vi "S4GUI_002.vi"(7 "Tab ObsEng":enum32{"Obs", "CCD modes", "Eng"}(tab)) -> ()   [LabVIEW 2018] (continued)
        n4615 = call "Write Instrument.lvclass.vi"("error in (no error)"=w11048, "Instrument.lvclass"=w11033, "S4ACS_GUI in"=w11035) -> ("error out"=w11029:errorcluster, "S4ACS_GUI out"=w11030:refnum<class "S4GUI.lvclass">)  [unwired: 7 in]
        n4616 = call "Read Instrument.lvclass.vi"("error in (no error)"=w11029, "S4ACS_GUI in"=w11030) -> ("error out"=w11098:errorcluster, "Instrument.lvclass"=w11099:refnum<class "Instrument.lvclass">, "S4ACS_GUI out"=w10945:refnum<class "S4GUI.lvclass">)  [unwired: 7 in]
        n4617 = call "Read WPSEL.vi"("error in (no error)"=w11098, "Instrument in"=w11099) -> ("error out"=w11095:errorcluster, "Opt_Selector.lvclass"=w11097:refnum<class "Opt_Selector.lvclass">, "Instrument out"=w11089:refnum<class "Instrument.lvclass">)  [unwired: 7 in]
        n4618 = call-dynamic "Read State Machine.vi"("error in (no error)"=w11095, "Device in"=w11097) -> ("error out"=w11094:errorcluster, "State Machine.lvclass"=w11087:refnum<class "State Machine.lvclass">, "Device out"=w11091:refnum<class "Opt_Selector.lvclass">)  [unwired: 7 in]
        n4619 = call "Next State.vi"("error in (no error)"=w11094, "New_State"=1, "State Machine in"=w11087) -> ("error out"=w11093:errorcluster, "State Machine out"=w11092:refnum<class "State Machine.lvclass">)  [unwired: 7 in]
        n4620 = call-dynamic "Write State Machine.vi"("error in (no error)"=w11093, "State Machine.lvclass"=w11092, "Device in"=w11091) -> ("error out"=w11088:errorcluster, "Device out"=w11090:refnum<class "Opt_Selector.lvclass">)  [unwired: 7 in]
        n4621 = call "Write WPSEL.vi"("error in (no error)"=w11088, "Opt_Selector.lvclass"=w11090, "Instrument in"=w11089) -> ("error out"=w11079:errorcluster, "Instrument out"=w11078:refnum<class "Instrument.lvclass">)  [unwired: 7 in]
        n4622 = call "Read ASEL.vi"("error in (no error)"=w11079, "Instrument in"=w11078) -> ("error out"=w11085:errorcluster, "Opt_Selector.lvclass"=w11076:refnum<class "Opt_Selector.lvclass">, "Instrument out"=w11077:refnum<class "Instrument.lvclass">)  [unwired: 7 in]
        n4623 = call-dynamic "Read State Machine.vi"("error in (no error)"=w11085, "Device in"=w11076) -> ("error out"=w11084:errorcluster, "State Machine.lvclass"=w11080:refnum<class "State Machine.lvclass">, "Device out"=w11075:refnum<class "Opt_Selector.lvclass">)  [unwired: 7 in]
        n4624 = call "Next State.vi"("error in (no error)"=w11084, "New_State"=1, "State Machine in"=w11080) -> ("error out"=w11083:errorcluster, "State Machine out"=w11082:refnum<class "State Machine.lvclass">)  [unwired: 7 in]
        n4625 = call-dynamic "Write State Machine.vi"("error in (no error)"=w11083, "State Machine.lvclass"=w11082, "Device in"=w11075) -> ("error out"=w11081:errorcluster, "Device out"=w11074:refnum<class "Opt_Selector.lvclass">)  [unwired: 7 in]
        n4626 = Concatenate Strings("SET WAVEPLATE:  WPSEL=" ("string"), w10924, " CALW=" ("string"), w10927) -> (w10937:string)
        n4627 = call "Write ASEL.vi"("error in (no error)"=w11081, "Opt_Selector.lvclass"=w11074, "Instrument in"=w11077) -> ("error out"=w11061:errorcluster, "Instrument out"=w11063:refnum<class "Instrument.lvclass">)  [unwired: 7 in]
        n4628 = call "Read CALW.vi"("error in (no error)"=w11061, "Instrument in"=w11063) -> ("error out"=w11071:errorcluster, "Opt_Selector.lvclass"=w11073:refnum<class "Opt_Selector.lvclass">, "Instrument out"=w11062:refnum<class "Instrument.lvclass">)  [unwired: 7 in]
        n4629 = call-dynamic "Read State Machine.vi"("error in (no error)"=w11071, "Device in"=w11073) -> ("error out"=w11070:errorcluster, "State Machine.lvclass"=w11064:refnum<class "State Machine.lvclass">, "Device out"=w11067:refnum<class "Opt_Selector.lvclass">)  [unwired: 7 in]
        n4630 = call "Next State.vi"("error in (no error)"=w11070, "New_State"=1, "State Machine in"=w11064) -> ("error out"=w11069:errorcluster, "State Machine out"=w11068:refnum<class "State Machine.lvclass">)  [unwired: 7 in]
        n4631 = call-dynamic "Write State Machine.vi"("error in (no error)"=w11069, "State Machine.lvclass"=w11068, "Device in"=w11067) -> ("error out"=w11065:errorcluster, "Device out"=w11066:refnum<class "Opt_Selector.lvclass">)  [unwired: 7 in]
        n4632 = property on="Lambda Selector" class="Ring (strict)"() -> ("RingText.Text"=w11060:string)  [unwired: 2 in, 2 out]
        n4633 = call "Write CALW.vi"("error in (no error)"=w11065, "Opt_Selector.lvclass"=w11066, "Instrument in"=w11062) -> ("error out"=w10944:errorcluster, "Instrument out"=w11059:refnum<class "Instrument.lvclass">)  [unwired: 7 in]
        n4634 = call-dynamic "Read mode EXPOSE.vi"("error in (no error)"=w10944, "S4GUI in"=w10945) -> ("error out"=w10943:errorcluster, "mode EXPOSE"=w10941:bool, "S4GUI out"=w10942:refnum<class "S4GUI.lvclass">)  [unwired: 7 in]
        n4635 = call-dynamic "Read sync.vi"("error in (no error)"=w10943, "S4ACS_GUI in"=w10942) -> ("error out"=w10961:errorcluster, "sync"=w10960:bool, "S4ACS_GUI out"=w10962:refnum<class "S4GUI.lvclass">)  [unwired: 7 in]
        n4636 = case shown="\"OFF\"" w11060 {
          selector: w11060 -> [w11307 _]
          tunnel: w11059 -> [w11311 w11329]
          tunnel: [w11310 w11329] -> w11058
          tunnel: [w11303 w11328] -> w10978
          tunnel: w10961 -> [w11309 w11328]
          tunnel: [w11300 w11324] -> w10973
          tunnel: w10960 -> [w11299 _]
          tunnel: w10941 -> [w11298 w11327]
          frame "OFF" {
            w11301 = u16 0 items=["OFF", "POLARIZER", "PINHOLE", "SHUTTER", "DEPOLARIZER"] ("Calibrator Selector 2")
            n4637 = call "Read CALW.vi"("error in (no error)"=w11309, "Instrument in"=w11311) -> ("error out"=w11314:errorcluster, "Opt_Selector.lvclass"=w11316:refnum<class "Opt_Selector.lvclass">, "Instrument out"=w11315:refnum<class "Instrument.lvclass">)  [unwired: 7 in]
            n4638 = call "Write target.vi"("error in (no error)"=w11314, "target"=0.0, "Optics in"=w11316) -> ("error out"=w11313:errorcluster, "Optics out"=w11317:refnum<class "Opt_Selector.lvclass">)  [unwired: 7 in]
            n4639 = call "Write target name.vi"("error in (no error)"=w11313, "target name"=w11307, "Optics in"=w11317) -> ("error out"=w11312:errorcluster, "Optics out"=w11318:refnum<class "Opt_Selector.lvclass">)  [unwired: 7 in]
            n4640 = call "Write CALW.vi"("error in (no error)"=w11312, "Opt_Selector.lvclass"=w11318, "Instrument in"=w11315) -> ("error out"=w11302:errorcluster, "Instrument out"=w11310:refnum<class "Instrument.lvclass">)  [unwired: 7 in]
            n4641 = property on="Calibrator Selector" class="Ring (strict)"(error in=w11302, "Value"=w11301, "DisabledEnum"=T12."Disabled and Grayed Out" ("Disabled")) -> (error out=w11304:errorcluster)  [unwired: 1 in, 1 out]
            n4642 = property on="Calibrator Selector" class="Ring (strict)"(error in=w11304, "RingText.Text"="OFF" ("Ring Text.Text")) -> (error out=w11303:errorcluster)  [unwired: 1 in, 1 out]
            n4643 = case shown="True" w11299 {
              tunnel: [u8 0 ("SHUTTER_MODE") w11321] -> w11300
              tunnel: w11298 -> [_ w11320]
              frame False {
                # "Fotom. & Async"
                # "Internal"
              }
              frame True {
                # "Ext. Start"
                # "Internal"
                # "Fotom. Sync. SEM exp mode"
                # "Fotom. Sync. COM exp mode"
                n4644 = Select(t=u8 0, s=w11320, f=u8 6 ("SHUTTER_MODE")) -> (s? t:f=w11321:u8)
              }
            }
          }
          frame Default {
            # "Polar. COM exp mode"
            # "Internal"
            # "Polar. SEM exp mode"
            # "Ext. Start"
            n4645 = Select(t=u8 0, s=w11327, f=u8 6 ("SHUTTER_MODE")) -> (s? t:f=w11324:u8)
          }
        }
        n4646 = call "Write Instrument.lvclass.vi"("error in (no error)"=w10978, "Instrument.lvclass"=w11058, "S4ACS_GUI in"=w10962) -> ("error out"=w10977:errorcluster, "S4ACS_GUI out"=w10966:refnum<class "S4GUI.lvclass">)  [unwired: 7 in]
        n4647 = call-dynamic "Read AcquisitionC.vi"("error in (no error)"=w10977, "S4ACS_GUI in"=w10966) -> ("error out"=w10988:errorcluster, "Acquisition.lvclass"=w10987:refnum<class "Acquisition.lvclass">)  [unwired: 7 in, 1 out]
        n4648 = call-dynamic "Read AcquisitionA.vi"("error in (no error)"=w10977, "S4ACS_GUI in"=w10966) -> ("error out"=w10991:errorcluster, "Acquisition.lvclass"=w10992:refnum<class "Acquisition.lvclass">)  [unwired: 7 in, 1 out]
        n4649 = call "Read AcquisitionB.vi"("error in (no error)"=w10977, "S4ACS_GUI in"=w10966) -> ("error out"=w10989:errorcluster, "Acquisition.lvclass"=w10990:refnum<class "Acquisition.lvclass">)  [unwired: 7 in, 1 out]
        n4650 = call-dynamic "Read AcquisitionD.vi"("error in (no error)"=w10977, "S4ACS_GUI in"=w10966) -> ("error out"=w10985:errorcluster, "Acquisition.lvclass"=w10986:refnum<class "Acquisition.lvclass">)  [unwired: 7 in, 1 out]
        n4651 = call "Read connection.vi"("error in (no error)"=w10988, "Server in"=w10987) -> ("error out"=w10994:errorcluster, "connection"=w10993:bool, "Server out"=w10995:refnum<class "Acquisition.lvclass">)  [unwired: 7 in]
        n4652 = call "Read connection.vi"("error in (no error)"=w10989, "Server in"=w10990) -> ("error out"=w10997:errorcluster, "connection"=w10996:bool, "Server out"=w10998:refnum<class "Acquisition.lvclass">)  [unwired: 7 in]
        n4653 = call "Read connection.vi"("error in (no error)"=w10985, "Server in"=w10986) -> ("error out"=w10974:errorcluster, "connection"=w10975:bool, "Server out"=w10976:refnum<class "Acquisition.lvclass">)  [unwired: 7 in]
        n4654 = call "Read connection.vi"("error in (no error)"=w10991, "Server in"=w10992) -> ("error out"=w11000:errorcluster, "connection"=w10999:bool, "Server out"=w11001:refnum<class "Acquisition.lvclass">)  [unwired: 7 in]
        n4655 = case shown="True" w10993 {
          tunnel: w10995 -> [w11165 w11170]
          tunnel: w10994 -> [w11164 w11169]
          tunnel: [w11165 w11168] -> w10980
          tunnel: [w11164 w11167] -> w10979
          tunnel: w10973 -> [_ w11166]
          frame False {
          }
          frame True {
            # "nome do arquivo .cfg"
            # "seção no arquivo .cfg"
            n4656 = call-dynamic "Read Channel.vi"("error in (no error)"=w11169, "Acquisition in"=w11170) -> ("error out"=w11174:errorcluster, "Channel.lvclass"=w11173:refnum<class "Channel.lvclass">, "Acquisition out"=w11172:refnum<class "Acquisition.lvclass">)  [unwired: 7 in]
            n4657 = call-dynamic "Read Interface.vi"("error in (no error)"=w11174, "Channel in"=w11173) -> ("error out"=w11181:errorcluster, "Interface.lvclass"=w11182:refnum<class "Interface.lvclass">, "Channel out"=w11171:refnum<class "Channel.lvclass">)  [unwired: 7 in]
            n4658 = call-dynamic "Get CCD_Config.vi"("error in (no error)"=w11181, "Interface in"=w11182) -> ("error out"=w11179:errorcluster, "output cluster"=w11178:T31, "Interface out"=w11183:refnum<class "Interface.lvclass">)  [unwired: 7 in]
            n4659 = Bundle By Name(cluster=w11178, "TRIGGER_MODE"=w11166) -> (w11180:T31)
            n4660 = call-dynamic "Set CCD_Config.vi"("error in (no error)"=w11179, "input cluster"=w11180, "Interface in"=w11183) -> ("error out"=w11177:errorcluster, "Interface out"=w11184:refnum<class "Interface.lvclass">)  [unwired: 7 in]
            n4661 = Flatten To String(anything=w11180, error in (no error)=w11177) -> (data string=w11175:string, error out=w11176:errorcluster)  [unwired: 2 in, 1 out]
            n4662 = call "Write flatted cluster.vi"("error in (no error)"=w11176, "flatted cluster"=w11175, "Interface in"=w11184) -> ("error out"=w11186:errorcluster, "Interface out"=w11185:refnum<class "Interface.lvclass">)  [unwired: 7 in]
            n4663 = call-dynamic "Write Interface.vi"("error in (no error)"=w11186, "Interface.lvclass"=w11185, "Channel in"=w11171) -> ("error out"=w11192:errorcluster, "Channel out"=w11193:refnum<class "Channel.lvclass">)  [unwired: 7 in]
            n4664 = call "Write section_name.vi"("error in (no error)"=w11192, "section_name"="CCD_ACS3", "Channel in"=w11193) -> ("error out"=w11190:errorcluster, "Channel out"=w11196:refnum<class "Channel.lvclass">)  [unwired: 7 in]
            n4665 = call-dynamic "save config.vi"("error in (no error)"=w11190, "file config"="lastsaved.cfg", "Channel in"=w11196) -> ("error out"=w11191:errorcluster, "Channel out"=w11197:refnum<class "Channel.lvclass">)  [unwired: 7 in]
            n4666 = call-dynamic "Read State Machine.vi"("error in (no error)"=w11191, "Device in"=w11197) -> ("error out"=w11187:errorcluster, "State Machine.lvclass"=w11199:refnum<class "State Machine.lvclass">, "Device out"=w11198:refnum<class "Channel.lvclass">)  [unwired: 7 in]
            n4667 = call-dynamic "Write State.vi"("error in (no error)"=w11187, "State"=60, "State Machine in"=w11199) -> ("error out"=w11188:errorcluster, "State Machine out"=w11200:refnum<class "State Machine.lvclass">)  [unwired: 7 in]
            n4668 = call-dynamic "Write State Machine.vi"("error in (no error)"=w11188, "State Machine.lvclass"=w11200, "Device in"=w11198) -> ("error out"=w11202:errorcluster, "Device out"=w11201:refnum<class "Channel.lvclass">)  [unwired: 7 in]
            n4669 = call-dynamic "Write Channel.vi"("error in (no error)"=w11202, "Channel.lvclass"=w11201, "Acquisition in"=w11172) -> ("error out"=w11167:errorcluster, "Acquisition out"=w11168:refnum<class "Acquisition.lvclass">)  [unwired: 7 in]
          }
        }
        n4670 = case shown="True" w10975 {
          tunnel: w10976 -> [w11126 w11131]
          tunnel: w10974 -> [w11125 w11130]
          tunnel: w10973 -> [_ w11129]
          tunnel: [w11126 w11128] -> w10972
          tunnel: [w11125 w11127] -> w10971
          frame False {
          }
          frame True {
            # "nome do arquivo .cfg"
            # "seção no arquivo .cfg"
            n4671 = call-dynamic "Read Channel.vi"("error in (no error)"=w11130, "Acquisition in"=w11131) -> ("error out"=w11160:errorcluster, "Channel.lvclass"=w11161:refnum<class "Channel.lvclass">, "Acquisition out"=w11162:refnum<class "Acquisition.lvclass">)  [unwired: 7 in]
            n4672 = call-dynamic "Read Interface.vi"("error in (no error)"=w11160, "Channel in"=w11161) -> ("error out"=w11153:errorcluster, "Interface.lvclass"=w11152:refnum<class "Interface.lvclass">, "Channel out"=w11163:refnum<class "Channel.lvclass">)  [unwired: 7 in]
            n4673 = call-dynamic "Get CCD_Config.vi"("error in (no error)"=w11153, "Interface in"=w11152) -> ("error out"=w11155:errorcluster, "output cluster"=w11156:T31, "Interface out"=w11151:refnum<class "Interface.lvclass">)  [unwired: 7 in]
            n4674 = Bundle By Name(cluster=w11156, "TRIGGER_MODE"=w11129) -> (w11154:T31)
            n4675 = call-dynamic "Set CCD_Config.vi"("error in (no error)"=w11155, "input cluster"=w11154, "Interface in"=w11151) -> ("error out"=w11157:errorcluster, "Interface out"=w11150:refnum<class "Interface.lvclass">)  [unwired: 7 in]
            n4676 = Flatten To String(anything=w11154, error in (no error)=w11157) -> (data string=w11159:string, error out=w11158:errorcluster)  [unwired: 2 in, 1 out]
            n4677 = call "Write flatted cluster.vi"("error in (no error)"=w11158, "flatted cluster"=w11159, "Interface in"=w11150) -> ("error out"=w11148:errorcluster, "Interface out"=w11149:refnum<class "Interface.lvclass">)  [unwired: 7 in]
            n4678 = call-dynamic "Write Interface.vi"("error in (no error)"=w11148, "Interface.lvclass"=w11149, "Channel in"=w11163) -> ("error out"=w11142:errorcluster, "Channel out"=w11141:refnum<class "Channel.lvclass">)  [unwired: 7 in]
            n4679 = call "Write section_name.vi"("error in (no error)"=w11142, "section_name"="CCD_ACS4", "Channel in"=w11141) -> ("error out"=w11144:errorcluster, "Channel out"=w11138:refnum<class "Channel.lvclass">)  [unwired: 7 in]
            n4680 = call-dynamic "save config.vi"("error in (no error)"=w11144, "file config"="lastsaved.cfg", "Channel in"=w11138) -> ("error out"=w11143:errorcluster, "Channel out"=w11137:refnum<class "Channel.lvclass">)  [unwired: 7 in]
            n4681 = call-dynamic "Read State Machine.vi"("error in (no error)"=w11143, "Device in"=w11137) -> ("error out"=w11147:errorcluster, "State Machine.lvclass"=w11135:refnum<class "State Machine.lvclass">, "Device out"=w11136:refnum<class "Channel.lvclass">)  [unwired: 7 in]
            n4682 = call-dynamic "Write State.vi"("error in (no error)"=w11147, "State"=60, "State Machine in"=w11135) -> ("error out"=w11146:errorcluster, "State Machine out"=w11134:refnum<class "State Machine.lvclass">)  [unwired: 7 in]
            n4683 = call-dynamic "Write State Machine.vi"("error in (no error)"=w11146, "State Machine.lvclass"=w11134, "Device in"=w11136) -> ("error out"=w11132:errorcluster, "Device out"=w11133:refnum<class "Channel.lvclass">)  [unwired: 7 in]
            n4684 = call-dynamic "Write Channel.vi"("error in (no error)"=w11132, "Channel.lvclass"=w11133, "Acquisition in"=w11162) -> ("error out"=w11127:errorcluster, "Acquisition out"=w11128:refnum<class "Acquisition.lvclass">)  [unwired: 7 in]
          }
        }
        n4685 = case shown="True" w10996 {
          tunnel: w10998 -> [w11204 w11209]
          tunnel: w10997 -> [w11203 w11208]
          tunnel: [w11204 w11207] -> w10982
          tunnel: [w11203 w11206] -> w10981
          tunnel: w10973 -> [_ w11205]
          frame False {
          }
          frame True {
            # "nome do arquivo .cfg"
            # "seção no arquivo .cfg"
            n4686 = call-dynamic "Read Channel.vi"("error in (no error)"=w11208, "Acquisition in"=w11209) -> ("error out"=w11213:errorcluster, "Channel.lvclass"=w11212:refnum<class "Channel.lvclass">, "Acquisition out"=w11211:refnum<class "Acquisition.lvclass">)  [unwired: 7 in]
            n4687 = call-dynamic "Read Interface.vi"("error in (no error)"=w11213, "Channel in"=w11212) -> ("error out"=w11220:errorcluster, "Interface.lvclass"=w11221:refnum<class "Interface.lvclass">, "Channel out"=w11210:refnum<class "Channel.lvclass">)  [unwired: 7 in]
            n4688 = call-dynamic "Get CCD_Config.vi"("error in (no error)"=w11220, "Interface in"=w11221) -> ("error out"=w11218:errorcluster, "output cluster"=w11217:T31, "Interface out"=w11222:refnum<class "Interface.lvclass">)  [unwired: 7 in]
            n4689 = Bundle By Name(cluster=w11217, "TRIGGER_MODE"=w11205) -> (w11219:T31)
            n4690 = call-dynamic "Set CCD_Config.vi"("error in (no error)"=w11218, "input cluster"=w11219, "Interface in"=w11222) -> ("error out"=w11216:errorcluster, "Interface out"=w11223:refnum<class "Interface.lvclass">)  [unwired: 7 in]
            n4691 = Flatten To String(anything=w11219, error in (no error)=w11216) -> (data string=w11214:string, error out=w11215:errorcluster)  [unwired: 2 in, 1 out]
            n4692 = call "Write flatted cluster.vi"("error in (no error)"=w11215, "flatted cluster"=w11214, "Interface in"=w11223) -> ("error out"=w11225:errorcluster, "Interface out"=w11224:refnum<class "Interface.lvclass">)  [unwired: 7 in]
            n4693 = call-dynamic "Write Interface.vi"("error in (no error)"=w11225, "Interface.lvclass"=w11224, "Channel in"=w11210) -> ("error out"=w11231:errorcluster, "Channel out"=w11232:refnum<class "Channel.lvclass">)  [unwired: 7 in]
            n4694 = call "Write section_name.vi"("error in (no error)"=w11231, "section_name"="CCD_ACS2", "Channel in"=w11232) -> ("error out"=w11229:errorcluster, "Channel out"=w11235:refnum<class "Channel.lvclass">)  [unwired: 7 in]
            n4695 = call-dynamic "save config.vi"("error in (no error)"=w11229, "file config"="lastsaved.cfg", "Channel in"=w11235) -> ("error out"=w11230:errorcluster, "Channel out"=w11236:refnum<class "Channel.lvclass">)  [unwired: 7 in]
            n4696 = call-dynamic "Read State Machine.vi"("error in (no error)"=w11230, "Device in"=w11236) -> ("error out"=w11226:errorcluster, "State Machine.lvclass"=w11238:refnum<class "State Machine.lvclass">, "Device out"=w11237:refnum<class "Channel.lvclass">)  [unwired: 7 in]
            n4697 = call-dynamic "Write State.vi"("error in (no error)"=w11226, "State"=60, "State Machine in"=w11238) -> ("error out"=w11227:errorcluster, "State Machine out"=w11239:refnum<class "State Machine.lvclass">)  [unwired: 7 in]
            n4698 = call-dynamic "Write State Machine.vi"("error in (no error)"=w11227, "State Machine.lvclass"=w11239, "Device in"=w11237) -> ("error out"=w11241:errorcluster, "Device out"=w11240:refnum<class "Channel.lvclass">)  [unwired: 7 in]
            n4699 = call-dynamic "Write Channel.vi"("error in (no error)"=w11241, "Channel.lvclass"=w11240, "Acquisition in"=w11211) -> ("error out"=w11206:errorcluster, "Acquisition out"=w11207:refnum<class "Acquisition.lvclass">)  [unwired: 7 in]
          }
        }
        n4700 = case shown="True" w10999 {
          tunnel: [w11242 w11276] -> w10983
          tunnel: [w11243 w11275] -> w10984
          tunnel: w11001 -> [w11243 w11246]
          tunnel: w11000 -> [w11242 w11245]
          tunnel: w10973 -> [_ w11244]
          frame False {
          }
          frame True {
            # "nome do arquivo .cfg"
            # "seção no arquivo .cfg"
            n4701 = call-dynamic "Read Channel.vi"("error in (no error)"=w11245, "Acquisition in"=w11246) -> ("error out"=w11277:errorcluster, "Channel.lvclass"=w11278:refnum<class "Channel.lvclass">, "Acquisition out"=w11279:refnum<class "Acquisition.lvclass">)  [unwired: 7 in]
            n4702 = call-dynamic "Read Interface.vi"("error in (no error)"=w11277, "Channel in"=w11278) -> ("error out"=w11268:errorcluster, "Interface.lvclass"=w11267:refnum<class "Interface.lvclass">, "Channel out"=w11280:refnum<class "Channel.lvclass">)  [unwired: 7 in]
            n4703 = call-dynamic "Get CCD_Config.vi"("error in (no error)"=w11268, "Interface in"=w11267) -> ("error out"=w11270:errorcluster, "output cluster"=w11271:T31, "Interface out"=w11266:refnum<class "Interface.lvclass">)  [unwired: 7 in]
            n4704 = Bundle By Name(cluster=w11271, "TRIGGER_MODE"=w11244) -> (w11269:T31)
            n4705 = call-dynamic "Set CCD_Config.vi"("error in (no error)"=w11270, "input cluster"=w11269, "Interface in"=w11266) -> ("error out"=w11272:errorcluster, "Interface out"=w11265:refnum<class "Interface.lvclass">)  [unwired: 7 in]
            n4706 = Flatten To String(anything=w11269, error in (no error)=w11272) -> (data string=w11274:string, error out=w11273:errorcluster)  [unwired: 2 in, 1 out]
            n4707 = call "Write flatted cluster.vi"("error in (no error)"=w11273, "flatted cluster"=w11274, "Interface in"=w11265) -> ("error out"=w11263:errorcluster, "Interface out"=w11264:refnum<class "Interface.lvclass">)  [unwired: 7 in]
            n4708 = call-dynamic "Write Interface.vi"("error in (no error)"=w11263, "Interface.lvclass"=w11264, "Channel in"=w11280) -> ("error out"=w11258:errorcluster, "Channel out"=w11257:refnum<class "Channel.lvclass">)  [unwired: 7 in]
            n4709 = call "Write section_name.vi"("error in (no error)"=w11258, "section_name"="CCD_ACS1", "Channel in"=w11257) -> ("error out"=w11259:errorcluster, "Channel out"=w11254:refnum<class "Channel.lvclass">)  [unwired: 7 in]
            n4710 = call-dynamic "save config.vi"("error in (no error)"=w11259, "file config"="lastsaved.cfg", "Channel in"=w11254) -> ("error out"=w11247:errorcluster, "Channel out"=w11248:refnum<class "Channel.lvclass">)  [unwired: 7 in]
            n4711 = call-dynamic "Read State Machine.vi"("error in (no error)"=w11247, "Device in"=w11248) -> ("error out"=w11262:errorcluster, "State Machine.lvclass"=w11252:refnum<class "State Machine.lvclass">, "Device out"=w11253:refnum<class "Channel.lvclass">)  [unwired: 7 in]
            n4712 = call-dynamic "Write State.vi"("error in (no error)"=w11262, "State"=60, "State Machine in"=w11252) -> ("error out"=w11261:errorcluster, "State Machine out"=w11251:refnum<class "State Machine.lvclass">)  [unwired: 7 in]
            n4713 = call-dynamic "Write State Machine.vi"("error in (no error)"=w11261, "State Machine.lvclass"=w11251, "Device in"=w11253) -> ("error out"=w11249:errorcluster, "Device out"=w11250:refnum<class "Channel.lvclass">)  [unwired: 7 in]
            n4714 = call-dynamic "Write Channel.vi"("error in (no error)"=w11249, "Channel.lvclass"=w11250, "Acquisition in"=w11279) -> ("error out"=w11276:errorcluster, "Acquisition out"=w11275:refnum<class "Acquisition.lvclass">)  [unwired: 7 in]
          }
        }
        n4715 = call-dynamic "Write AcquisitionA.vi"("error in (no error)"=w10983, "Acquisition.lvclass"=w10984, "S4ACS_GUI in"=w10966) -> ("error out"=w10970:errorcluster, "S4ACS_GUI out"=w10965:refnum<class "S4GUI.lvclass">)  [unwired: 7 in]
        n4716 = call "Write AcquisitionB.vi"("error in (no error)"=w10981, "Acquisition.lvclass"=w10982, "S4ACS_GUI in"=w10965) -> ("error out"=w10969:errorcluster, "S4ACS_GUI out"=w10964:refnum<class "S4GUI.lvclass">)  [unwired: 7 in]
        n4717 = call-dynamic "Write AcquisitionC.vi"("error in (no error)"=w10979, "Acquisition.lvclass"=w10980, "S4ACS_GUI in"=w10964) -> ("error out"=w10968:errorcluster, "S4ACS_GUI out"=w10963:refnum<class "S4GUI.lvclass">)  [unwired: 7 in]
        n4718 = call-dynamic "Write AcquisitionD.vi"("error in (no error)"=w10971, "Acquisition.lvclass"=w10972, "S4ACS_GUI in"=w10963) -> ("error out"=w10967:errorcluster, "S4ACS_GUI out"=w10947:refnum<class "S4GUI.lvclass">)  [unwired: 7 in]
        n4719 = Merge Errors(w10970, w10969, w10968, w10967) -> (w10946:errorcluster)
        n4720 = call "Read Instrument.lvclass.vi"("error in (no error)"=w10946, "S4ACS_GUI in"=w10947) -> ("error out"=w10952:errorcluster, "Instrument.lvclass"=w10951:refnum<class "Instrument.lvclass">, "S4ACS_GUI out"=w10948:refnum<class "S4GUI.lvclass">)  [unwired: 7 in]
        n4721 = call "Read ASEL.vi"("error in (no error)"=w10952, "Instrument in"=w10951) -> ("error out"=w10959:errorcluster, "Opt_Selector.lvclass"=w10958:refnum<class "Opt_Selector.lvclass">, "Instrument out"=w10957:refnum<class "Instrument.lvclass">)  [unwired: 7 in]
        n4722 = call "Read target name.vi"("error in (no error)"=w10959, "Optics in"=w10958) -> ("error out"=w10955:errorcluster, "target name"=w10935:string, "Optics out"=w10956:refnum<class "Opt_Selector.lvclass">)  [unwired: 7 in]
        n4723 = call "Write ASEL.vi"("error in (no error)"=w10955, "Opt_Selector.lvclass"=w10956, "Instrument in"=w10957) -> ("error out"=w10954:errorcluster, "Instrument out"=w10950:refnum<class "Instrument.lvclass">)  [unwired: 7 in]
        n4724 = Concatenate Strings(w10937, " ASEL=" ("string"), w10935) -> (w10932:string)
        n4725 = case shown="\"ON\"" w10935 {
          tunnel: w10954 -> [w11101 w11112]
          tunnel: [w11101 w11108] -> w10953
          tunnel: w10950 -> [w11100 w11113]
          tunnel: [w11100 w11109] -> w10949
          frame Default {
          }
          frame "ON" {
            n4726 = call "Read WPROT.vi"("error in (no error)"=w11112, "Instrument in"=w11113) -> ("error out"=w11104:errorcluster, "Opt_Selector.lvclass"=w11111:refnum<class "Opt_Selector.lvclass">, "Instrument out"=w11110:refnum<class "Instrument.lvclass">)  [unwired: 7 in]
            n4727 = call-dynamic "Read sequencia.vi"("error in (no error)"=w11104, "Opt_Selector in"=w11111) -> ("error out"=w11103:errorcluster, "sequencia"=w11107:u16, "Opt_Selector out"=w11106:refnum<class "Opt_Selector.lvclass">)  [unwired: 7 in]
            n4728 = case shown="0" w11107 {
              tunnel: w11106 -> [w11115 w11124]
              tunnel: [w11115 w11120] -> w11105
              tunnel: w11103 -> [w11114 w11123]
              tunnel: [w11114 w11118] -> w11102
              frame Default {
              }
              frame 0 {
                n4729 = call-dynamic "Write sequencia.vi"("error in (no error)"=w11123, "sequencia"=u16 1, "Opt_Selector in"=w11124) -> ("error out"=w11119:errorcluster, "Opt_Selector out"=w11121:refnum<class "Opt_Selector.lvclass">)  [unwired: 7 in]
                n4730 = local write "P0"(TRUE ("P0")) -> ()
                n4731 = call-dynamic "Write sequencia_ant.vi"("error in (no error)"=w11119, "sequencia_ant"=u16 1, "Opt_Selector in"=w11121) -> ("error out"=w11118:errorcluster, "Opt_Selector out"=w11120:refnum<class "Opt_Selector.lvclass">)  [unwired: 7 in]
              }
            }
            n4732 = call "Write WPROT.vi"("error in (no error)"=w11102, "Opt_Selector.lvclass"=w11105, "Instrument in"=w11110) -> ("error out"=w11108:errorcluster, "Instrument out"=w11109:refnum<class "Instrument.lvclass">)  [unwired: 7 in]
          }
        }
        n4733 = call "Write Instrument.lvclass.vi"("error in (no error)"=w10953, "Instrument.lvclass"=w10949, "S4ACS_GUI in"=w10948) -> ("error out"=w10933:errorcluster, "S4ACS_GUI out"=w10934:refnum<class "S4GUI.lvclass">)  [unwired: 7 in]
        n4734 = call-dynamic "Write User Event.vi"("error in (no error)"=w10933, "User Event"=w10932, "S4GUI in"=w10934) -> ("error out"=w10930:errorcluster, "S4GUI out"=w10931:refnum<class "S4GUI.lvclass">)  [unwired: 7 in]
      }
      event "Init mode": Value Change {
        n4735 = event-data() -> ()  [unwired: 1 in, 4 out]
        n4736 = call-dynamic "Write User Event.vi"("error in (no error)"=w11333, "User Event"="INIT INSTRUMENT CLICKED", "S4GUI in"=w11334) -> ("error out"=w11331:errorcluster, "S4GUI out"=w11332:refnum<class "S4GUI.lvclass">)  [unwired: 7 in]
        n4737 = call-dynamic "Read Obs_state.vi"("error in (no error)"=w11331, "S4ACS_GUI in"=w11332) -> ("error out"=w11335:errorcluster, "Obs_state"=w11337:u32, "S4ACS_GUI out"=w11338:refnum<class "S4GUI.lvclass">)  [unwired: 7 in]
        n4738 = In Range and Coerce(upper limit=u32 226, x=w11337, lower limit=u32 220 ("upper limit")) -> (In Range?=w11336:bool)  [unwired: 1 out]
        n4739 = case shown="True" w11336 {
          tunnel: [w11346 w11354] -> w11342
          tunnel: [w11345 w11352] -> w11341
          tunnel: w11335 -> [w11344 w11353]
          tunnel: w11338 -> [w11343 w11355]
          frame False {
            n4740 = call-dynamic "Write sync.vi"("error in (no error)"=w11344, "sync"=TRUE, "S4ACS_GUI in"=w11343) -> ("error out"=w11348:errorcluster, "S4ACS_GUI out"=w11347:refnum<class "S4GUI.lvclass">)  [unwired: 7 in]
            n4741 = call-dynamic "Write Obs_state.vi"("error in (no error)"=w11348, "Obs_state"=u32 220, "S4ACS_GUI in"=w11347) -> ("error out"=w11345:errorcluster, "S4ACS_GUI out"=w11346:refnum<class "S4GUI.lvclass">)  [unwired: 7 in]
          }
          frame True {
            n4742 = call-dynamic "Write Obs_state.vi"("error in (no error)"=w11353, "Obs_state"=u32 0, "S4ACS_GUI in"=w11355) -> ("error out"=w11352:errorcluster, "S4ACS_GUI out"=w11354:refnum<class "S4GUI.lvclass">)  [unwired: 7 in]
          }
        }
      }
      event "exit": Value Change {
        n4743 = event-data() -> ()  [unwired: 1 in, 4 out]
        n4744 = call-dynamic "Read Obs_state.vi"("error in (no error)"=w11359, "S4ACS_GUI in"=w11360) -> ("error out"=w11357:errorcluster, "Obs_state"=w11361:u32, "S4ACS_GUI out"=w11358:refnum<class "S4GUI.lvclass">)  [unwired: 7 in]
        n4745 = In Range and Coerce(upper limit=u32 239, x=w11361, lower limit=u32 230 ("upper limit")) -> (In Range?=w11356:bool)  [unwired: 1 out]
        n4746 = case shown="False" w11356 {
          tunnel: [w11374 w11494] -> w11365
          tunnel: [w11373 w11493] -> w11364
          tunnel: w11358 -> [w11367 w11494]
          tunnel: w11357 -> [w11366 w11493]
          frame False {
            n4747 = call "Read Instrument.lvclass.vi"("error in (no error)"=w11366, "S4ACS_GUI in"=w11367) -> ("error out"=w11368:errorcluster, "Instrument.lvclass"=w11370:refnum<class "Instrument.lvclass">, "S4ACS_GUI out"=w11372:refnum<class "S4GUI.lvclass">)  [unwired: 7 in]
            n4748 = call-dynamic "Read operational.vi"("error in (no error)"=w11368, "Server in"=w11370) -> ("error out"=w11371:errorcluster, "operational"=w11369:bool)  [unwired: 7 in, 1 out]
            n4749 = case shown="False" w11369 {
              tunnel: [w11381 w11438] -> w11374
              tunnel: [w11380 w11437] -> w11373
              tunnel: w11372 -> [w11376 w11440]
              tunnel: w11371 -> [w11375 w11439]
              frame False {
                # "S4ICS not operational: only ACS parking can \nbe allowed, depending on its status..."
                n4750 = call-dynamic "VerifyAcqStatus.vi"("error in (no error)"=w11375, "S4GUI in"=w11376) -> ("error out"=w11377:errorcluster, "idle"=w11379:bool, "S4GUI out"=w11378:refnum<class "S4GUI.lvclass">)  [unwired: 6 in, 1 out]
                n4751 = case shown="True" w11379 {
                  tunnel: w11377 -> [w11390 w11409]
                  tunnel: w11378 -> [w11391 w11408]
                  tunnel: [w11384 w11407] -> w11381
                  tunnel: [w11383 w11406] -> w11380
                  frame False {
                    # "Acquisition in progress..."
                    n4752 = Two Button Dialog(message="Parking not possible.\nAre you sure to quit?", 2:"Yes" ("T button name (\"OK\")")) -> (T button?=w11387:bool)  [unwired: 1 in]
                    n4753 = case shown="False" w11387 {
                      tunnel: [w11394 w11398] -> w11386
                      tunnel: w11391 -> [w11394 w11399]
                      tunnel: w11390 -> [w11393 w11397]
                      tunnel: [w11393 w11396] -> w11385
                      tunnel: ["EXIT CLICKED \nWITH NO PARKING \nPOSSIBLE. EXIT\nCANCELLED. " ("T button name (\"OK\")") "EXIT CLICKED WITH\nNO PARKING POSSIBLE. EXIT" ("T button name (\"OK\")")] -> w11382
                      frame False {
                        # "NO (cancel)"
                      }
                      frame True {
                        # "YES"
                        n4754 = call-dynamic "Write exit.vi"("error in (no error)"=w11397, "exit"=TRUE, "S4GUI in"=w11399) -> ("error out"=w11396:errorcluster, "S4GUI out"=w11398:refnum<class "S4GUI.lvclass">)  [unwired: 7 in]
                      }
                    }
                    n4755 = call-dynamic "Write User Event.vi"("error in (no error)"=w11385, "User Event"=w11382, "S4GUI in"=w11386) -> ("error out"=w11383:errorcluster, "S4GUI out"=w11384:refnum<class "S4GUI.lvclass">)  [unwired: 7 in]
                  }
                  frame True {
                    # "No acquisition in progress."
                    n4756 = call <vilib>:"Three Button Dialog.vi"("Right Button Text (\"Cancel\")"="Cancel" ("Right Button Text (\"Cancel\")"), "Center Button Text (\"No\")"="NO" ("F button name (\"Cancel\")"), "Left Button Text (\"Yes\")"="YES" ("T button name (\"OK\")"), "message"="Instrument parking not possible.\nPark acquisition system before exiting?") -> ("Which Button?"=w11404:T34)  [unwired: 7 in]
                    n4757 = case shown="\"Left Button\"" w11404 {
                      tunnel: w11409 -> [w11416 w11420 w11429]
                      tunnel: w11408 -> [w11415 w11421 w11428]
                      tunnel: [w11412 w11419 w11425] -> w11407
                      tunnel: [w11410 w11418 w11423] -> w11406
                      frame "Center Button" {
                        # "NO"
                        n4758 = call-dynamic "Write exit.vi"("error in (no error)"=w11416, "exit"=TRUE, "S4GUI in"=w11415) -> ("error out"=w11411:errorcluster, "S4GUI out"=w11413:refnum<class "S4GUI.lvclass">)  [unwired: 7 in]
                        n4759 = call-dynamic "Write User Event.vi"("error in (no error)"=w11411, "User Event"="EXIT APP CLICKED WITH NO PARKING.", "S4GUI in"=w11413) -> ("error out"=w11410:errorcluster, "S4GUI out"=w11412:refnum<class "S4GUI.lvclass">)  [unwired: 7 in]
                      }
                      frame "Right Button", Default {
                        # "CANCEL"
                        n4760 = call-dynamic "Write User Event.vi"("error in (no error)"=w11420, "User Event"="EXIT APP CLICKED, BUT CANCELLED BY USER.", "S4GUI in"=w11421) -> ("error out"=w11418:errorcluster, "S4GUI out"=w11419:refnum<class "S4GUI.lvclass">)  [unwired: 7 in]
                      }
                      frame "Left Button" {
                        # "YES"
                        n4761 = call-dynamic "Write sync.vi"("error in (no error)"=w11429, "sync"=TRUE, "S4ACS_GUI in"=w11428) -> ("error out"=w11431:errorcluster, "S4ACS_GUI out"=w11430:refnum<class "S4GUI.lvclass">)  [unwired: 7 in]
                        n4762 = call-dynamic "Write Obs_state.vi"("error in (no error)"=w11431, "Obs_state"=u32 232, "S4ACS_GUI in"=w11430) -> ("error out"=w11424:errorcluster, "S4ACS_GUI out"=w11426:refnum<class "S4GUI.lvclass">)  [unwired: 7 in]
                        n4763 = call-dynamic "Write User Event.vi"("error in (no error)"=w11424, "User Event"="EXIT APP CLICKED AND ONLY ACS PARKING PROCEDURE DONE.", "S4GUI in"=w11426) -> ("error out"=w11423:errorcluster, "S4GUI out"=w11425:refnum<class "S4GUI.lvclass">)  [unwired: 7 in]
                      }
                    }
                  }
                }
              }
              frame True {
                # "S4ICS operational: Instrument parking allowed \nand verifying ACS channels status..."
                n4764 = call-dynamic "VerifyAcqStatus.vi"("error in (no error)"=w11439, "S4GUI in"=w11440) -> ("error out"=w11435:errorcluster, "idle"=w11434:bool, "S4GUI out"=w11436:refnum<class "S4GUI.lvclass">)  [unwired: 6 in, 1 out]
                n4765 = case shown="True" w11434 {
                  tunnel: [w11444 w11468] -> w11438
                  tunnel: [w11443 w11467] -> w11437
                  tunnel: w11436 -> [w11442 w11461]
                  tunnel: w11435 -> [w11441 w11460]
                  frame False {
                    # "Acquisition in progress..."
                    n4766 = Two Button Dialog(message="Parking not possible.\nAre you sure to quit?", 2:"Yes" ("T button name (\"OK\")")) -> (T button?=w11448:bool)  [unwired: 1 in]
                    n4767 = case shown="True" w11448 {
                      tunnel: [w11453 w11457] -> w11447
                      tunnel: w11442 -> [w11453 w11458]
                      tunnel: w11441 -> [w11452 w11456]
                      tunnel: [w11452 w11455] -> w11446
                      tunnel: ["EXIT CLICKED \nWITH NO PARKING \nPOSSIBLE. EXIT\nCANCELLED. " ("T button name (\"OK\")") "EXIT CLICKED WITH\nNO PARKING POSSIBLE. EXIT" ("T button name (\"OK\")")] -> w11445
                      frame False {
                        # "NO (cancel)"
                      }
                      frame True {
                        # "YES"
                        n4768 = call-dynamic "Write exit.vi"("error in (no error)"=w11456, "exit"=TRUE, "S4GUI in"=w11458) -> ("error out"=w11455:errorcluster, "S4GUI out"=w11457:refnum<class "S4GUI.lvclass">)  [unwired: 7 in]
                      }
                    }
                    n4769 = call-dynamic "Write User Event.vi"("error in (no error)"=w11446, "User Event"=w11445, "S4GUI in"=w11447) -> ("error out"=w11443:errorcluster, "S4GUI out"=w11444:refnum<class "S4GUI.lvclass">)  [unwired: 7 in]
                  }
                  frame True {
                    # "Acquisition system in IDLE state."
                    n4770 = call <vilib>:"Three Button Dialog.vi"("Right Button Text (\"Cancel\")"="Cancel" ("Right Button Text (\"Cancel\")"), "Center Button Text (\"No\")"="NO" ("F button name (\"Cancel\")"), "Left Button Text (\"Yes\")"="YES" ("T button name (\"OK\")"), "message"="Park before exiting?") -> ("Which Button?"=w11463:T34)  [unwired: 7 in]
                    n4771 = case shown="\"Right Button\", Default" w11463 {
                      tunnel: w11460 -> [w11475 w11479 w11489]
                      tunnel: w11461 -> [w11474 w11480 w11488]
                      tunnel: [w11471 w11478 w11485] -> w11468
                      tunnel: [w11469 w11477 w11483] -> w11467
                      frame "Center Button" {
                        # "NO"
                        n4772 = call-dynamic "Write exit.vi"("error in (no error)"=w11475, "exit"=TRUE, "S4GUI in"=w11474) -> ("error out"=w11470:errorcluster, "S4GUI out"=w11472:refnum<class "S4GUI.lvclass">)  [unwired: 7 in]
                        n4773 = call-dynamic "Write User Event.vi"("error in (no error)"=w11470, "User Event"="EXIT APP CLICKED WITH NO PARKING.", "S4GUI in"=w11472) -> ("error out"=w11469:errorcluster, "S4GUI out"=w11471:refnum<class "S4GUI.lvclass">)  [unwired: 7 in]
                      }
                      frame "Right Button", Default {
                        # "CANCEL"
                        n4774 = call-dynamic "Write User Event.vi"("error in (no error)"=w11479, "User Event"="EXIT APP CLICKED, BUT CANCELLED BY USER.", "S4GUI in"=w11480) -> ("error out"=w11477:errorcluster, "S4GUI out"=w11478:refnum<class "S4GUI.lvclass">)  [unwired: 7 in]
                      }
                      frame "Left Button" {
                        # "YES"
                        n4775 = call-dynamic "Write sync.vi"("error in (no error)"=w11489, "sync"=TRUE, "S4ACS_GUI in"=w11488) -> ("error out"=w11491:errorcluster, "S4ACS_GUI out"=w11490:refnum<class "S4GUI.lvclass">)  [unwired: 7 in]
                        n4776 = call-dynamic "Write Obs_state.vi"("error in (no error)"=w11491, "Obs_state"=u32 230, "S4ACS_GUI in"=w11490) -> ("error out"=w11484:errorcluster, "S4ACS_GUI out"=w11486:refnum<class "S4GUI.lvclass">)  [unwired: 7 in]
                        n4777 = call-dynamic "Write User Event.vi"("error in (no error)"=w11484, "User Event"="EXIT APP CLICKED AND PARKING PROCEDURE DONE.", "S4GUI in"=w11486) -> ("error out"=w11483:errorcluster, "S4GUI out"=w11485:refnum<class "S4GUI.lvclass">)  [unwired: 7 in]
                      }
                    }
                  }
                }
              }
            }
          }
          frame True {
            # "Parking already in progress..."
          }
        }
      }
      event "WPSEL_stop": Value Change {
        n4778 = event-data() -> ()  [unwired: 1 in, 4 out]
        n4779 = call "Read Instrument.lvclass.vi"("error in (no error)"=w11513, "S4ACS_GUI in"=w11514) -> ("error out"=w11511:errorcluster, "Instrument.lvclass"=w11512:refnum<class "Instrument.lvclass">, "S4ACS_GUI out"=w11498:refnum<class "S4GUI.lvclass">)  [unwired: 7 in]
        n4780 = call "Read WPSEL.vi"("error in (no error)"=w11511, "Instrument in"=w11512) -> ("error out"=w11507:errorcluster, "Opt_Selector.lvclass"=w11510:refnum<class "Opt_Selector.lvclass">, "Instrument out"=w11501:refnum<class "Instrument.lvclass">)  [unwired: 7 in]
        n4781 = call-dynamic "Read State Machine.vi"("error in (no error)"=w11507, "Device in"=w11510) -> ("error out"=w11506:errorcluster, "State Machine.lvclass"=w11509:refnum<class "State Machine.lvclass">, "Device out"=w11503:refnum<class "Opt_Selector.lvclass">)  [unwired: 7 in]
        n4782 = call "Next State.vi"("error in (no error)"=w11506, "New_State"=10, "State Machine in"=w11509) -> ("error out"=w11505:errorcluster, "State Machine out"=w11504:refnum<class "State Machine.lvclass">)  [unwired: 7 in]
        n4783 = call-dynamic "Write State Machine.vi"("error in (no error)"=w11505, "State Machine.lvclass"=w11504, "Device in"=w11503) -> ("error out"=w11500:errorcluster, "Device out"=w11502:refnum<class "Opt_Selector.lvclass">)  [unwired: 7 in]
        n4784 = call "Write WPSEL.vi"("error in (no error)"=w11500, "Opt_Selector.lvclass"=w11502, "Instrument in"=w11501) -> ("error out"=w11497:errorcluster, "Instrument out"=w11499:refnum<class "Instrument.lvclass">)  [unwired: 7 in]
        n4785 = call "Write Instrument.lvclass.vi"("error in (no error)"=w11497, "Instrument.lvclass"=w11499, "S4ACS_GUI in"=w11498) -> ("error out"=w11496:errorcluster, "S4ACS_GUI out"=w11495:refnum<class "S4GUI.lvclass">)  [unwired: 7 in]
      }
      event "WPSEL_init": Value Change {
        n4786 = event-data() -> ()  [unwired: 1 in, 4 out]
        n4787 = call "Read Instrument.lvclass.vi"("error in (no error)"=w11533, "S4ACS_GUI in"=w11534) -> ("error out"=w11531:errorcluster, "Instrument.lvclass"=w11532:refnum<class "Instrument.lvclass">, "S4ACS_GUI out"=w11518:refnum<class "S4GUI.lvclass">)  [unwired: 7 in]
        n4788 = call "Read WPSEL.vi"("error in (no error)"=w11531, "Instrument in"=w11532) -> ("error out"=w11527:errorcluster, "Opt_Selector.lvclass"=w11530:refnum<class "Opt_Selector.lvclass">, "Instrument out"=w11521:refnum<class "Instrument.lvclass">)  [unwired: 7 in]
        n4789 = call-dynamic "Read State Machine.vi"("error in (no error)"=w11527, "Device in"=w11530) -> ("error out"=w11526:errorcluster, "State Machine.lvclass"=w11529:refnum<class "State Machine.lvclass">, "Device out"=w11523:refnum<class "Opt_Selector.lvclass">)  [unwired: 7 in]
        n4790 = call "Next State.vi"("error in (no error)"=w11526, "New_State"=30, "State Machine in"=w11529) -> ("error out"=w11525:errorcluster, "State Machine out"=w11524:refnum<class "State Machine.lvclass">)  [unwired: 7 in]
        n4791 = call-dynamic "Write State Machine.vi"("error in (no error)"=w11525, "State Machine.lvclass"=w11524, "Device in"=w11523) -> ("error out"=w11520:errorcluster, "Device out"=w11522:refnum<class "Opt_Selector.lvclass">)  [unwired: 7 in]
        n4792 = call "Write WPSEL.vi"("error in (no error)"=w11520, "Opt_Selector.lvclass"=w11522, "Instrument in"=w11521) -> ("error out"=w11517:errorcluster, "Instrument out"=w11519:refnum<class "Instrument.lvclass">)  [unwired: 7 in]
        n4793 = call "Write Instrument.lvclass.vi"("error in (no error)"=w11517, "Instrument.lvclass"=w11519, "S4ACS_GUI in"=w11518) -> ("error out"=w11516:errorcluster, "S4ACS_GUI out"=w11515:refnum<class "S4GUI.lvclass">)  [unwired: 7 in]
      }
      event "GMIR_target": Value Change {
        n4794 = event-data() -> ("NewVal"=w11544:dbl)  [unwired: 1 in, 3 out]
        n4795 = call "Read Instrument.lvclass.vi"("error in (no error)"=w11548, "S4ACS_GUI in"=w11549) -> ("error out"=w11546:errorcluster, "Instrument.lvclass"=w11547:refnum<class "Instrument.lvclass">, "S4ACS_GUI out"=w11538:refnum<class "S4GUI.lvclass">)  [unwired: 7 in]
        n4796 = call "Read GMIR.vi"("error in (no error)"=w11546, "Instrument in"=w11547) -> ("error out"=w11543:errorcluster, "Opt_Continuous.lvclass"=w11545:refnum<class "Opt_Continuous.lvclass">, "Instrument out"=w11541:refnum<class "Instrument.lvclass">)  [unwired: 7 in]
        n4797 = call "Write target.vi"("error in (no error)"=w11543, "target"=w11544, "Optics in"=w11545) -> ("error out"=w11540:errorcluster, "Optics out"=w11542:refnum<class "Opt_Continuous.lvclass">)  [unwired: 7 in]
        n4798 = call "Write GMIR.vi"("error in (no error)"=w11540, "Opt_Continuous.lvclass"=w11542, "Instrument in"=w11541) -> ("error out"=w11537:errorcluster, "Instrument out"=w11539:refnum<class "Instrument.lvclass">)  [unwired: 7 in]
        n4799 = call "Write Instrument.lvclass.vi"("error in (no error)"=w11537, "Instrument.lvclass"=w11539, "S4ACS_GUI in"=w11538) -> ("error out"=w11536:errorcluster, "S4ACS_GUI out"=w11535:refnum<class "S4GUI.lvclass">)  [unwired: 7 in]
      }
      event "GMIR_set": Value Change {
        n4800 = event-data() -> ()  [unwired: 1 in, 4 out]
        n4801 = call "Read Instrument.lvclass.vi"("error in (no error)"=w11568, "S4ACS_GUI in"=w11569) -> ("error out"=w11566:errorcluster, "Instrument.lvclass"=w11567:refnum<class "Instrument.lvclass">, "S4ACS_GUI out"=w11555:refnum<class "S4GUI.lvclass">)  [unwired: 7 in]
        n4802 = call "Read GMIR.vi"("error in (no error)"=w11566, "Instrument in"=w11567) -> ("error out"=w11563:errorcluster, "Opt_Continuous.lvclass"=w11565:refnum<class "Opt_Continuous.lvclass">, "Instrument out"=w11557:refnum<class "Instrument.lvclass">)  [unwired: 7 in]
        n4803 = call-dynamic "Read State Machine.vi"("error in (no error)"=w11563, "Device in"=w11565) -> ("error out"=w11562:errorcluster, "State Machine.lvclass"=w11553:refnum<class "State Machine.lvclass">, "Device out"=w11559:refnum<class "Opt_Continuous.lvclass">)  [unwired: 7 in]
        n4804 = call "Next State.vi"("error in (no error)"=w11562, "New_State"=1, "State Machine in"=w11553) -> ("error out"=w11561:errorcluster, "State Machine out"=w11560:refnum<class "State Machine.lvclass">)  [unwired: 7 in]
        n4805 = call-dynamic "Write State Machine.vi"("error in (no error)"=w11561, "State Machine.lvclass"=w11560, "Device in"=w11559) -> ("error out"=w11556:errorcluster, "Device out"=w11558:refnum<class "Opt_Continuous.lvclass">)  [unwired: 7 in]
        n4806 = call "Write GMIR.vi"("error in (no error)"=w11556, "Opt_Continuous.lvclass"=w11558, "Instrument in"=w11557) -> ("error out"=w11550:errorcluster, "Instrument out"=w11551:refnum<class "Instrument.lvclass">)  [unwired: 7 in]
        n4807 = call "Write Instrument.lvclass.vi"("error in (no error)"=w11550, "Instrument.lvclass"=w11551, "S4ACS_GUI in"=w11555) -> ("error out"=w11554:errorcluster, "S4ACS_GUI out"=w11552:refnum<class "S4GUI.lvclass">)  [unwired: 7 in]
      }
      event "GMIR_stop": Value Change {
        n4808 = event-data() -> ()  [unwired: 1 in, 4 out]
        n4809 = call "Read Instrument.lvclass.vi"("error in (no error)"=w11588, "S4ACS_GUI in"=w11589) -> ("error out"=w11586:errorcluster, "Instrument.lvclass"=w11587:refnum<class "Instrument.lvclass">, "S4ACS_GUI out"=w11573:refnum<class "S4GUI.lvclass">)  [unwired: 7 in]
        n4810 = call "Read GMIR.vi"("error in (no error)"=w11586, "Instrument in"=w11587) -> ("error out"=w11582:errorcluster, "Opt_Continuous.lvclass"=w11585:refnum<class "Opt_Continuous.lvclass">, "Instrument out"=w11576:refnum<class "Instrument.lvclass">)  [unwired: 7 in]
        n4811 = call-dynamic "Read State Machine.vi"("error in (no error)"=w11582, "Device in"=w11585) -> ("error out"=w11581:errorcluster, "State Machine.lvclass"=w11584:refnum<class "State Machine.lvclass">, "Device out"=w11578:refnum<class "Opt_Continuous.lvclass">)  [unwired: 7 in]
        n4812 = call "Next State.vi"("error in (no error)"=w11581, "New_State"=10, "State Machine in"=w11584) -> ("error out"=w11580:errorcluster, "State Machine out"=w11579:refnum<class "State Machine.lvclass">)  [unwired: 7 in]
        n4813 = call-dynamic "Write State Machine.vi"("error in (no error)"=w11580, "State Machine.lvclass"=w11579, "Device in"=w11578) -> ("error out"=w11575:errorcluster, "Device out"=w11577:refnum<class "Opt_Continuous.lvclass">)  [unwired: 7 in]
        n4814 = call "Write GMIR.vi"("error in (no error)"=w11575, "Opt_Continuous.lvclass"=w11577, "Instrument in"=w11576) -> ("error out"=w11572:errorcluster, "Instrument out"=w11574:refnum<class "Instrument.lvclass">)  [unwired: 7 in]
        n4815 = call "Write Instrument.lvclass.vi"("error in (no error)"=w11572, "Instrument.lvclass"=w11574, "S4ACS_GUI in"=w11573) -> ("error out"=w11571:errorcluster, "S4ACS_GUI out"=w11570:refnum<class "S4GUI.lvclass">)  [unwired: 7 in]
      }
      event "GMIR_init": Value Change {
        n4816 = event-data() -> ()  [unwired: 1 in, 4 out]
        n4817 = call "Read Instrument.lvclass.vi"("error in (no error)"=w11608, "S4ACS_GUI in"=w11609) -> ("error out"=w11606:errorcluster, "Instrument.lvclass"=w11607:refnum<class "Instrument.lvclass">, "S4ACS_GUI out"=w11593:refnum<class "S4GUI.lvclass">)  [unwired: 7 in]
        n4818 = call "Read GMIR.vi"("error in (no error)"=w11606, "Instrument in"=w11607) -> ("error out"=w11602:errorcluster, "Opt_Continuous.lvclass"=w11605:refnum<class "Opt_Continuous.lvclass">, "Instrument out"=w11596:refnum<class "Instrument.lvclass">)  [unwired: 7 in]
        n4819 = call-dynamic "Read State Machine.vi"("error in (no error)"=w11602, "Device in"=w11605) -> ("error out"=w11601:errorcluster, "State Machine.lvclass"=w11604:refnum<class "State Machine.lvclass">, "Device out"=w11598:refnum<class "Opt_Continuous.lvclass">)  [unwired: 7 in]
        n4820 = call "Next State.vi"("error in (no error)"=w11601, "New_State"=30, "State Machine in"=w11604) -> ("error out"=w11600:errorcluster, "State Machine out"=w11599:refnum<class "State Machine.lvclass">)  [unwired: 7 in]
